vi "Controle Moteurv2.vi"(8 "error in (no error)":errorcluster, 11 "Port COM":refnum<visa-resource-name>="COM4") -> (0 "error out":errorcluster)   [LabVIEW 2019]
doc: "Ce VI est une interface utilisateur qui permet à l'usager d'interagir avec le contrôlleur de moteur ST5-Q"
uses:
  <vilib>/Utility/error.llb/DialogType.ctl
panel:
  out "CW Limit":bool
  out "CCW Limit":bool
  out "Alarme":u32
  in  "Update":bool
  in  "Clr Alarm":bool
  out "Status":T1
  in  "Résolution Pas":dbl
  in  "Facteur Dir":bool
  in  "Facteur Pas":dbl=1500.0
  in  "Save":bool
  in  "Accél Max":dbl=0.167 caption="Accélération Max (Tour/s/s)" min=0.167 max=5461.167 step=0.167 format="%#.3g"
  in  "Stop":bool
  in  "Relatif":bool=TRUE caption="Relatif/Absolu\n(Absolu)"
  in  "Origine":bool
  in  "Direction":bool=TRUE
  in  "Déplacement":dbl caption="Position (trou)" min=-100.0 max=100.0 step=0.0001 format="%#.3g"
  in  "Décél":dbl=0.167 caption="Décélération \n(Tour/s/s)" min=0.167 max=5461.167 step=0.167 format="%#.3g"
  in  "Accél":dbl=0.167 caption="Accélération \n(Tour/s/s)" min=0.167 max=5461.167 step=0.167 format="%#.3g"
  out "Réponse":string
  in  "Commande":string
  in  "Envoyer":bool
  in  "Vitesse":dbl=0.08399999999999999 caption="Vitesse (Tour/s)" min=0.0042 max=133.3333 step=0.0042 format="%#.4g"
  in  "Quitter":bool
  # "Paramètres du moteur"
  # "Contrôle du moteur"
  # "Commande Manuel"
  # "Relatif"
  # "Absolu"
  # "Descendre(H)"
  # "Monter (AH)"
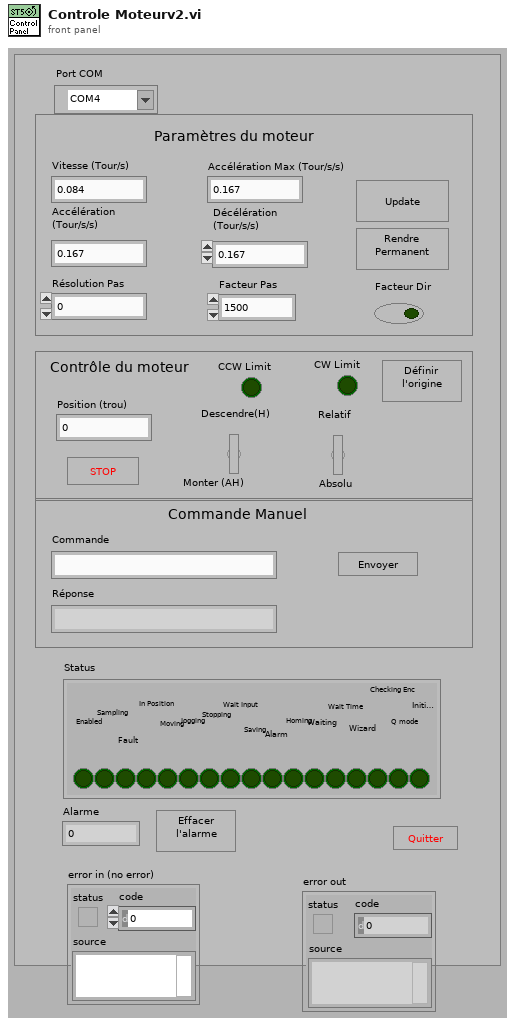
[diagram p1: front panel]
types:
  T1 = cluster{"Enabled":bool, "Sampling":bool, "Fault":bool, "In Position":bool, "Moving":bool, "Jogging":bool, "Stopping":bool, "Wait Input":bool, "Saving":bool, "Alarm":bool, "Homing":bool, "Waiting":bool, "Wait Time":bool, "Wizard":bool, "Checking Enc":bool, "Q mode":bool, "Initializing":bool}
  T2 = typedef "DialogType.ctl" = u16
  T3 = cluster{"Vitesse (Tour/s)":dbl, "Accél":dbl, "Décél":dbl, "Accél Max":dbl, "Idle Current (A) ":dbl}
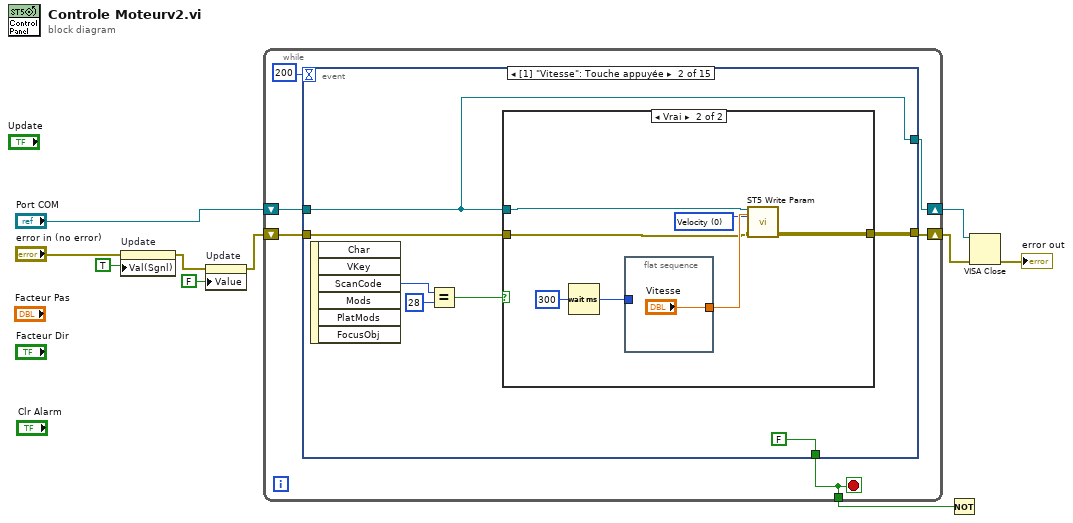
[diagram p0: block diagram]
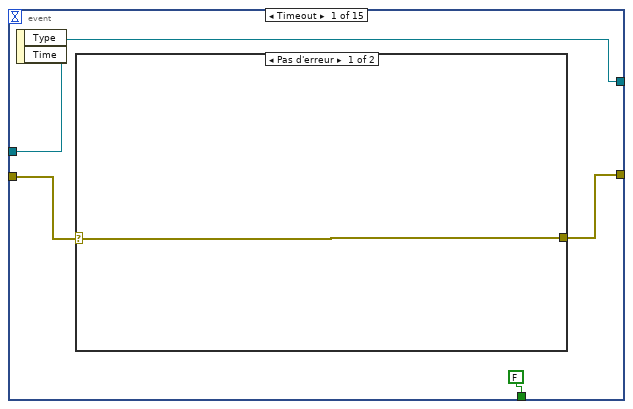
[diagram p2: hidden frame]
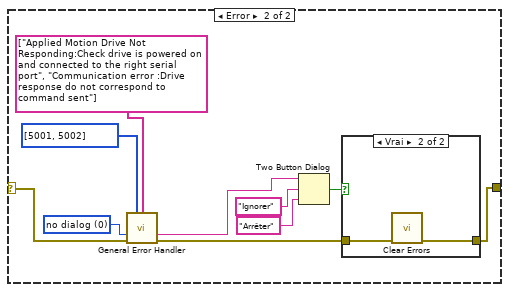
[diagram p3: hidden frame]
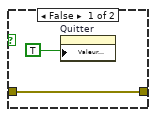
[diagram p4: hidden frame]
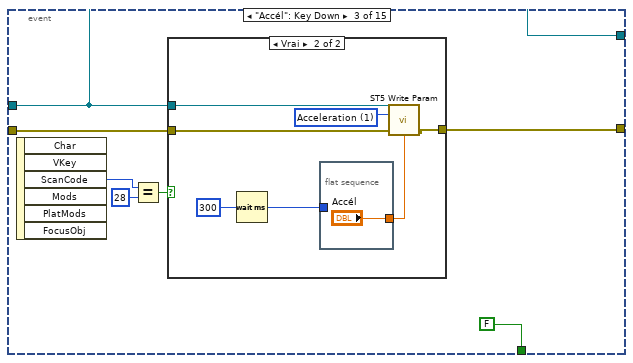
[diagram p6: hidden frame]
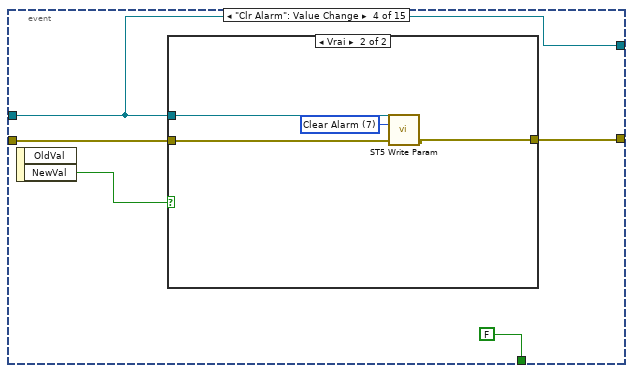
[diagram p8: hidden frame]
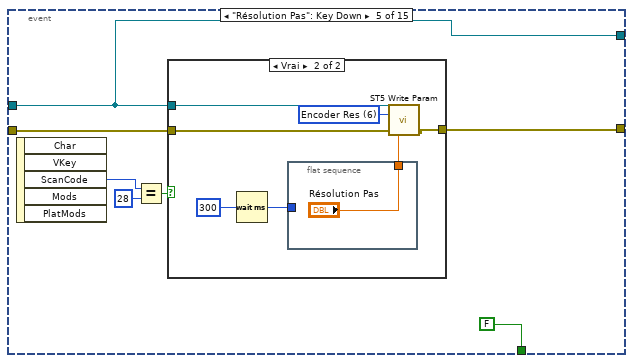
[diagram p10: hidden frame]
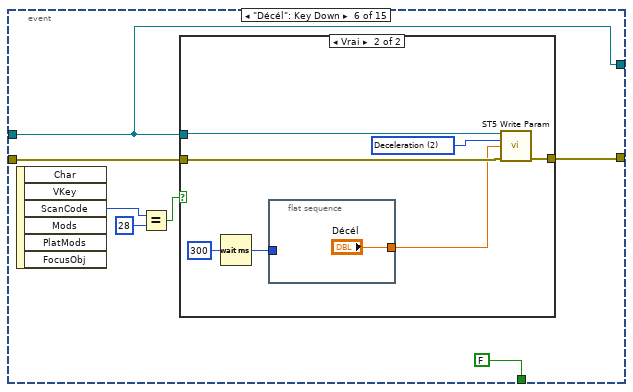
[diagram p12: hidden frame]
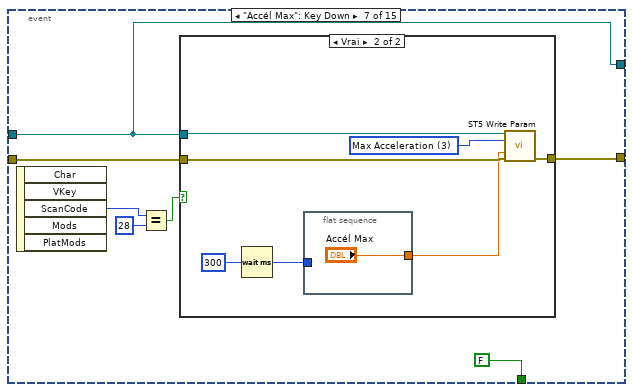
[diagram p14: hidden frame]
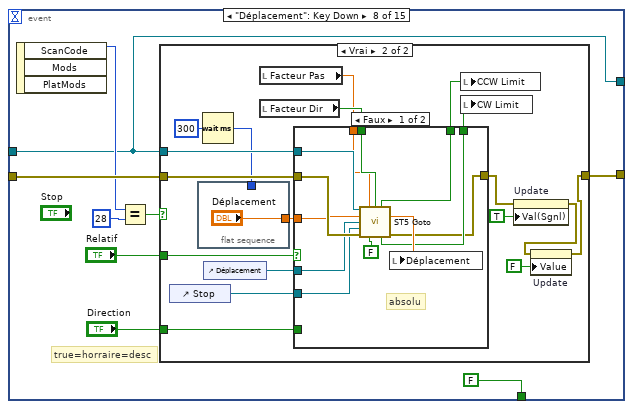
[diagram p16: hidden frame]
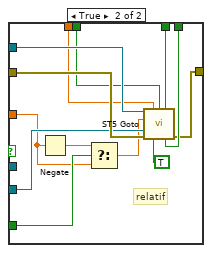
[diagram p18: hidden frame]
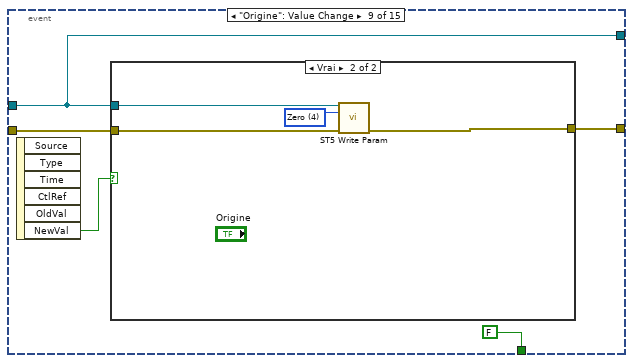
[diagram p19: hidden frame]
diagram:
  n1 = property on="Update" class="Bool (strict)"(error in="error in (no error)", "Val(Sgnl)"=TRUE ("Valeur (Signalisation)")) -> (error out=w2:errorcluster)  [unwired: 1 in, 1 out]
  n2 = property on="Update" class="Bool (strict)"(error in=w2, "Value"=FALSE ("Update")) -> (error out=w1:errorcluster)  [unwired: 1 in, 1 out]
  n3 = while {
    shift-right: [w15] -> w8
    shift-left: w1 -> [w16]
    tunnel: [w12] -> w10
    shift-right: [w11] -> w4
    shift-left: "Port COM" -> [w13]
    stop <- w12 stop-if-true
    n4 = event shown="[1] \"Vitesse\": Touche appuyée" {
      selector: _ -> [_ _ _ _ _ _ _ _ _ _ _ _ _ _ _]
      dyn-events: _ -> [_ _ _ _ _ _ _ _ _ _ _ _ _ _ _]
      timeout: 200 -> [_ _ _ _ _ _ _ _ _ _ _ _ _ _ _]
      tunnel: w16 -> [w20 w40 w56 w72 w84 w98 w114 w132 w184 w192 w201 w224 w244 _ _]
      tunnel: [w19 w39 w55 w71 w83 w97 w113 w131 w183 w191 w200 w240 w243 _ _] -> w15
      tunnel: w13 -> [w17 w37 w53 w68 w79 w94 w110 w126 w180 w190 w199 _ w241 w252 w254]
      tunnel: [FALSE ("Discard?") FALSE ("Discard?") FALSE ("Discard?") FALSE ("Discard?") FALSE ("Discard?") FALSE ("Discard?") FALSE ("Discard?") FALSE ("Discard?") FALSE ("Discard?") _ _ _ FALSE ("Discard?") w253 TRUE ("Discard?")] -> w12
      tunnel: [w17 w37 w53 w68 w79 w94 w110 w126 w180 w190 w199 w238 w241 w252 w254] -> w11
      event Timeout {
        n5 = event-data() -> ()  [unwired: 1 in, 2 out]
        n6 = case shown="Pas d'erreur" w20 {
          selector: w20 -> [w21 w25]
          tunnel: [w21 w26] -> w19
          frame No Error {
          }
          frame Error {
            w28 = T2 0 items=["no dialog", "OK message", "continue or stop message", "OK message + warnings", "continue/stop + warnings"] ("type of dialog (OK msg:1)")
            n7 = call <vilib>:"General Error Handler.vi"("[user-defined codes]"=i32[] [5001, 5002], "[user-defined descriptions]"=string[] ["Applied Motion Drive Not Responding:Check drive is powered on and connected to the right serial port", "Communication error :Drive response do not correspond to command sent"], "type of dialog (OK msg:1)"=w28, "error in (no error)"=w25) -> ("message"=w22:string, "error out"=w27:errorcluster)  [unwired: 7 in, 3 out]
            n8 = Two Button Dialog(message=w22, 1:"Arrêter" ("F button name (\"Cancel\")"), 2:"Ignorer" ("T button name (\"OK\")")) -> (T button?=w31:bool)
            n9 = case shown="Vrai" w31 {
              tunnel: w27 -> [w33 w34]
              tunnel: [w33 w35] -> w26
              frame False {
                n10 = property on="Quitter" class="Bool (strict)"("Valeur (Signalisation)"=TRUE ("Value (Signaling)")) -> ()  [unwired: 2 in, 2 out]
              }
              frame True {
                n11 = call <vilib>:"Clear Errors.vi"("error in (no error)"=w34) -> ("error out"=w35:errorcluster)  [unwired: 5 in, 1 out]
              }
            }
          }
        }
      }
      event "Vitesse": Key Down {
        n12 = event-data() -> ("ScanCode"=w36:i16)  [unwired: 1 in, 5 out]
        n13 = Equal?(x=w36, y=i16 28) -> (x = y?=w41:bool)
        n14 = case shown="Vrai" w41 {
          tunnel: w37 -> [_ w45]
          tunnel: w40 -> [w43 w46]
          tunnel: [w43 w50] -> w39
          frame False {
          }
          frame True {
            w48 = u16 0 items=["Velocity", "Acceleration", "Deceleration", "Max Acceleration", "Zero", "Save"] ("Parameters")
            n15 = Wait (ms)(milliseconds to wait=u32 300 ("attente (ms)")) -> (millisecond timer value=w44:u32)
            n16 = flat-sequence {
              tunnel: ["Vitesse"] -> w49
              tunnel: w44 -> [_]
              frame #0 {
              }
            }
            n17 = call <userlib>:"ST5 Write Param.vi"("Port COM"=w45, "Vitesse"=w49, "Parameters"=w48, "error in (no error)"=w46) -> ("error out"=w50:errorcluster)  [unwired: 10 in, 1 out]
          }
        }
      }
      event "Accél": Key Down {
        n18 = event-data() -> ("ScanCode"=w52:i16)  [unwired: 1 in, 5 out]
        n19 = Equal?(x=w52, y=i16 28) -> (x = y?=w57:bool)
        n20 = case shown="Vrai" w57 {
          tunnel: w53 -> [_ w64]
          tunnel: w56 -> [w59 w66]
          tunnel: [w59 w65] -> w55
          frame False {
          }
          frame True {
            w62 = u16 1 items=["Velocity", "Acceleration", "Deceleration", "Max Acceleration", "Zero", "Save"] ("Parameters")
            n21 = Wait (ms)(milliseconds to wait=u32 300 ("attente (ms)")) -> (millisecond timer value=w60:u32)
            n22 = flat-sequence {
              tunnel: ["Accél"] -> w63
              tunnel: w60 -> [_]
              frame #0 {
              }
            }
            n23 = call <userlib>:"ST5 Write Param.vi"("Port COM"=w64, "Accél"=w63, "Parameters"=w62, "error in (no error)"=w66) -> ("error out"=w65:errorcluster)  [unwired: 10 in, 1 out]
          }
        }
      }
      event "Clr Alarm": Value Change {
        n24 = event-data() -> ("NewVal"=w69:bool)  [unwired: 1 in, 1 out]
        n25 = case shown="Vrai" w69 {
          tunnel: w68 -> [_ w75]
          tunnel: w72 -> [w73 w77]
          tunnel: [w73 w76] -> w71
          frame False {
          }
          frame True {
            w74 = u16 7 items=["Velocity", "Acceleration", "Deceleration", "Max Acceleration", "Zero", "Save", "Encoder Res", "Clear Alarm"] ("Parameters")
            n26 = call <userlib>:"ST5 Write Param.vi"("Port COM"=w75, "Parameters"=w74, "error in (no error)"=w77) -> ("error out"=w76:errorcluster)  [unwired: 11 in, 1 out]
          }
        }
      }
      event "Résolution Pas": Key Down {
        n27 = event-data() -> ("ScanCode"=w78:i16)  [unwired: 1 in, 4 out]
        n28 = Equal?(x=w78, y=i16 28) -> (x = y?=w80:bool)
        n29 = case shown="Vrai" w80 {
          tunnel: w79 -> [_ w90]
          tunnel: w84 -> [w85 w92]
          tunnel: [w85 w91] -> w83
          frame False {
          }
          frame True {
            w87 = u16 6 items=["Velocity", "Acceleration", "Deceleration", "Max Acceleration", "Zero", "Save", "Encoder Res", "Clear Alarm"] ("Parameters")
            n30 = Wait (ms)(milliseconds to wait=u32 300 ("attente (ms)")) -> (millisecond timer value=w88:u32)
            n31 = flat-sequence {
              tunnel: w88 -> [_]
              tunnel: ["Résolution Pas"] -> w86
              frame #0 {
              }
            }
            n32 = call <userlib>:"ST5 Write Param.vi"("Port COM"=w90, "Parameters"=w87, "error in (no error)"=w92, "Microstep Res(Pas/Tour)"=w86) -> ("error out"=w91:errorcluster)  [unwired: 10 in, 1 out]
          }
        }
      }
      event "Décél": Key Down {
        n33 = event-data() -> ("ScanCode"=w95:i16)  [unwired: 1 in, 5 out]
        n34 = Equal?(x=w95, y=i16 28) -> (x = y?=w99:bool)
        n35 = case shown="Vrai" w99 {
          tunnel: w94 -> [_ w107]
          tunnel: w98 -> [w101 w108]
          tunnel: [w101 w106] -> w97
          frame False {
          }
          frame True {
            w105 = u16 2 items=["Velocity", "Acceleration", "Deceleration", "Max Acceleration", "Zero", "Save"] ("Parameters")
            n36 = Wait (ms)(milliseconds to wait=u32 300 ("attente (ms)")) -> (millisecond timer value=w103:u32)
            n37 = flat-sequence {
              tunnel: w103 -> [_]
              tunnel: ["Décél"] -> w102
              frame #0 {
              }
            }
            n38 = call <userlib>:"ST5 Write Param.vi"("Port COM"=w107, "Parameters"=w105, "Décél"=w102, "error in (no error)"=w108) -> ("error out"=w106:errorcluster)  [unwired: 10 in, 1 out]
          }
        }
      }
      event "Accél Max": Key Down {
        n39 = event-data() -> ("ScanCode"=w111:i16)  [unwired: 1 in, 4 out]
        n40 = Equal?(x=w111, y=i16 28) -> (x = y?=w115:bool)
        n41 = case shown="Vrai" w115 {
          tunnel: w110 -> [_ w123]
          tunnel: w114 -> [w117 w124]
          tunnel: [w117 w122] -> w113
          frame False {
          }
          frame True {
            w121 = u16 3 items=["Velocity", "Acceleration", "Deceleration", "Max Acceleration", "Zero", "Save"] ("Parameters")
            n42 = Wait (ms)(milliseconds to wait=u32 300 ("attente (ms)")) -> (millisecond timer value=w118:u32)
            n43 = flat-sequence {
              tunnel: ["Accél Max"] -> w120
              tunnel: w118 -> [_]
              frame #0 {
              }
            }
            n44 = call <userlib>:"ST5 Write Param.vi"("Port COM"=w123, "Parameters"=w121, "Accél Max"=w120, "error in (no error)"=w124) -> ("error out"=w122:errorcluster)  [unwired: 10 in, 1 out]
          }
        }
      }
      event "Déplacement": Key Down {
        # "true=horraire=desc"
        n45 = event-data() -> ("ScanCode"=w128:i16)  [unwired: 1 in, 2 out]
        n46 = Equal?(x=w128, y=i16 28) -> (x = y?=w133:bool)
        n47 = case shown="Vrai" w133 {
          tunnel: w126 -> [_ w152]
          tunnel: w132 -> [w135 w153]
          tunnel: [w135 w136] -> w131
          tunnel: "Direction" -> [_ w151]
          tunnel: "Relatif" -> [_ w150]
          frame False {
          }
          frame True {
            n48 = control-ref of="Stop"() -> (w149:refnum<vi>)
            n49 = flat-sequence {
              tunnel: ["Déplacement"] -> w148
              tunnel: w146 -> [_]
              frame #0 {
              }
            }
            n50 = Wait (ms)(milliseconds to wait=u32 300 ("attente (ms)")) -> (millisecond timer value=w146:u32)
            n51 = control-ref of="Déplacement"() -> (w143:refnum<vi>)
            n52 = local read "Facteur Pas"() -> (w144:dbl)
            n53 = local read "Facteur Dir"() -> (w145:bool)
            n54 = case shown="Faux" w150 {
              tunnel: [w155 w167] -> w139
              tunnel: w153 -> [w165 w178]
              tunnel: w152 -> [w166 w179]
              tunnel: w151 -> [_ w174]
              tunnel: w149 -> [w162 w177]
              tunnel: w148 -> [w161 w172]
              tunnel: w145 -> [w160 w170]
              tunnel: w144 -> [w159 w171]
              tunnel: w143 -> [w158 _]
              tunnel: [w157 w169] -> w142
              tunnel: [w156 w168] -> w141
              frame False {
                # "absolu"
                n55 = call <userlib>:"ST5 Goto.vi"("Port COM"=w166, "Facteur Pas"=w159, "Facteur Dir"=w160, "Position"=w161, "PositionRef"=w158, "Ext Stop Ref"=w162, "error in (no error)"=w165, "Relatif"=FALSE) -> ("CCW Limit"=w157:bool, "Position Out"=w164:dbl, "CW Limit"=w156:bool, "error out"=w155:errorcluster)  [unwired: 1 in, 3 out]
                n56 = local write "Déplacement"(w164) -> ()
              }
              frame True {
                # "relatif"
                n57 = Negate(x=w172) -> (-x=w173:dbl)
                n58 = Select(t=w173, s=w174, f=w172) -> (s? t:f=w176:dbl)
                n59 = call <userlib>:"ST5 Goto.vi"("Port COM"=w179, "Facteur Pas"=w171, "Facteur Dir"=w170, "Position"=w176, "Ext Stop Ref"=w177, "error in (no error)"=w178, "Relatif"=TRUE) -> ("CCW Limit"=w169:bool, "CW Limit"=w168:bool, "error out"=w167:errorcluster)  [unwired: 2 in, 4 out]
              }
            }
            n60 = local write "CCW Limit"(w142) -> ()
            n61 = local write "CW Limit"(w141) -> ()
            n62 = property on="Update" class="Bool (strict)"(error in=w139, "Val(Sgnl)"=TRUE ("Valeur (Signalisation)")) -> (error out=w137:errorcluster)  [unwired: 1 in, 1 out]
            n63 = property on="Update" class="Bool (strict)"(error in=w137, "Value"=FALSE ("Update")) -> (error out=w136:errorcluster)  [unwired: 1 in, 1 out]
          }
        }
      }
      event "Origine": Value Change {
        n64 = event-data() -> ("NewVal"=w181:bool)  [unwired: 1 in, 5 out]
        n65 = case shown="Vrai" w181 {
          tunnel: w184 -> [w185 w188]
          tunnel: w180 -> [_ w186]
          tunnel: [w185 w189] -> w183
          frame False {
          }
          frame True {
            w187 = u16 4 items=["Velocity", "Acceleration", "Deceleration", "Max Acceleration", "Zero", "Save"] ("Parameters")
            n66 = call <userlib>:"ST5 Write Param.vi"("Port COM"=w186, "Parameters"=w187, "error in (no error)"=w188) -> ("error out"=w189:errorcluster)  [unwired: 11 in, 1 out]
          }
        }
      }
      event "Save": Value Change {
        n67 = event-data() -> ("NewVal"=w193:bool)  [unwired: 1 in, 5 out]
        n68 = case shown="Vrai" w193 {
          tunnel: w190 -> [_ w198]
          tunnel: w192 -> [w194 w197]
          tunnel: [w194 w196] -> w191
          frame False {
          }
          frame True {
            w195 = u16 5 items=["Velocity", "Acceleration", "Deceleration", "Max Acceleration", "Zero", "Save"] ("Parameters")
            n69 = call <userlib>:"ST5 Write Param.vi"("Port COM"=w198, "Parameters"=w195, "error in (no error)"=w197) -> ("error out"=w196:errorcluster)  [unwired: 11 in, 1 out]
          }
        }
      }
      event "Update": Value Change {
        n70 = event-data() -> ("NewVal"=w202:bool)  [unwired: 1 in, 5 out]
        n71 = case shown="Faux" w202 {
          tunnel: w199 -> [_ w211]
          tunnel: w201 -> [w203 w210]
          tunnel: [w203 w212] -> w200
          frame False {
          }
          frame True {
            w220 = u16 0 items=["All", "Velocity", "Acceleration", "Deceleration", "Max Acceleration", "Position"] ("Parameters")
            n72 = local read "Facteur Pas"() -> (w222:dbl)
            n73 = local read "Facteur Dir"() -> (w221:bool)
            n74 = call <userlib>:"ST5 Read Param.vi"("Facteur Dir"=w221, "error in (no error)"=w210, "Facteur Pas"=w222, "Parameters"=w220, "Port COM"=w211) -> ("error out"=w212:errorcluster, "Status"=→"Status":T1, "Position"=w219:dbl, "Speed Par"=w218:T3, "Résolution Pas"=w213:dbl, "Alarme"=w208:u32)  [unwired: 1 out]
            "Alarme" <- w208
            n75 = Number To Boolean Array(number=w208) -> (Boolean array=w207:bool[])
            n76 = Unbundle By Name(w218) -> ("Vitesse (Tour/s)"=w217:dbl, "Accél"=w216:dbl, "Décél"=w215:dbl, "Accél Max"=w214:dbl)
            n77 = Index Array(array=w207, index #1=1 ("indice")) -> (element #1=→"CCW Limit":bool, element #2=→"CW Limit":bool)  [unwired: 1 in]
            n78 = local write "Résolution Pas"(w213) -> ()
            n79 = local write "Déplacement"(w219) -> ()
            n80 = local write "Vitesse"(w217) -> ()
            n81 = local write "Accél"(w216) -> ()
            n82 = local write "Décél"(w215) -> ()
            n83 = local write "Accél Max"(w214) -> ()
          }
        }
      }
      event "Port COM": Value Change {
        w234 = u16 0 items=["All", "Velocity", "Acceleration", "Deceleration", "Max Acceleration", "Position"] ("Parameters")
        n84 = event-data() -> ("OldVal"=w225:refnum<visa-resource-name>, "NewVal"=w239:refnum<visa-resource-name>)  [unwired: 1 in, 4 out]
        n85 = VISA Close(VISA resource name=w225, error in (no error)=w224) -> (error out=w223:errorcluster)
        n86 = local read "Facteur Pas"() -> (w237:dbl)
        n87 = local read "Facteur Dir"() -> (w236:bool)
        n88 = call <userlib>:"ST5 Read Param.vi"("Facteur Dir"=w236, "error in (no error)"=w223, "Facteur Pas"=w237, "Parameters"=w234, "Port COM"=w239) -> ("error out"=w240:errorcluster, "Status"=w235:T1, "Position"=w233:dbl, "Port COM Out"=w238:refnum<visa-resource-name>, "Speed Par"=w232:T3, "Résolution Pas"=w227:dbl, "Alarme"=w226:u32)
        n89 = Unbundle By Name(w232) -> ("Vitesse (Tour/s)"=w231:dbl, "Accél"=w230:dbl, "Décél"=w229:dbl, "Accél Max"=w228:dbl)
        n90 = local write "Résolution Pas"(w227) -> ()
        n91 = local write "Déplacement"(w233) -> ()
        n92 = local write "Alarme"(w226) -> ()
        n93 = local write "Status"(w235) -> ()
        n94 = local write "Vitesse"(w231) -> ()
        n95 = local write "Accél"(w230) -> ()
        n96 = local write "Décél"(w229) -> ()
        n97 = local write "Accél Max"(w228) -> ()
      }
      event "Envoyer": Value Change {
        n98 = event-data() -> ("NewVal"=w245:bool)  [unwired: 1 in]
        n99 = case shown="Vrai" w245 {
          tunnel: w244 -> [w246 w250]
          tunnel: [w246 w248] -> w243
          tunnel: w241 -> [_ w251]
          frame False {
          }
          frame True {
            n100 = call <userlib>:"Commande ST5V2.vi"("error in (no error)"=w250, "Commande"="Commande", "Port COM"=w251) -> ("error out"=w248:errorcluster, "Réponse"=→"Réponse":string)  [unwired: 1 in, 2 out]
          }
        }
      }
      event Panel Close? {
        w253 = TRUE ("Discard?")
        n101 = event-data() -> ()  [unwired: 1 in, 4 out]
        n102 = event-data("Discard?"=w253) -> ()  [unwired: 1 in, 1 out]
      }
      event "Quitter": Value Change {
        n103 = event-data() -> ()  [unwired: 1 in, 6 out]
      }
    }
  }
  n104 = Not(x=w10) -> ()  [unwired: 1 out]
  n105 = VISA Close(VISA resource name=w4, error in (no error)=w8) -> (error out=→"error out":errorcluster)
